vi "AdaptorControl01.vi"() -> ()   [LabVIEW 2011]
panel:
  in  "Local":bool
  in  "stop":bool
  out "Close active":bool
  out "Auto active":bool
  out "Open active":bool
  out "Hold active":bool
  out "Message":string
  out "D active":bool
  out "A active":bool
  out "B active":bool
  out "C active":bool
  in  "v":bool
  in  "^":bool
  in  "Mode":bool
  in  "Zero":bool
  out "Angle":string
  out "Pressure":string
  in  "D":bool
  in  "C":bool
  in  "B":bool
  in  "A":bool
  in  "Close":bool
  in  "Hold":bool
  in  "Open":bool
  in  "Auto":bool
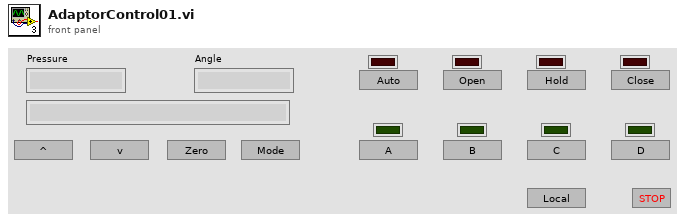
[diagram p1: front panel]
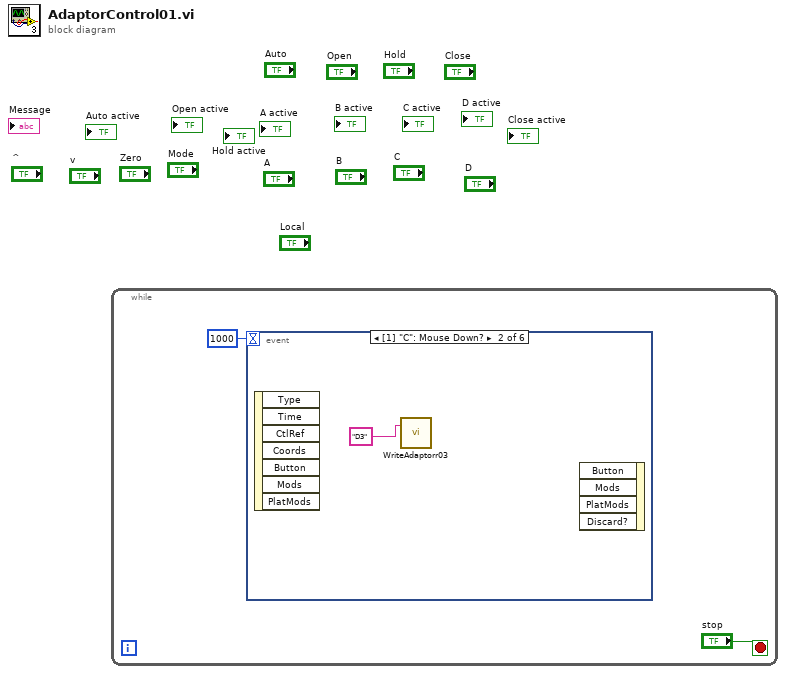
[diagram p0: block diagram]
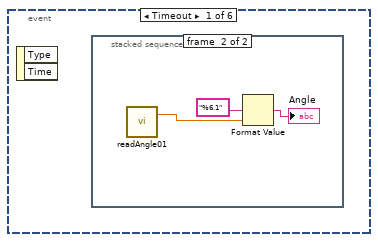
[diagram p2: hidden frame]
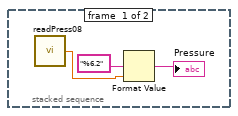
[diagram p3: hidden frame]
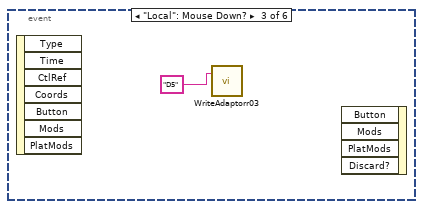
[diagram p4: hidden frame]
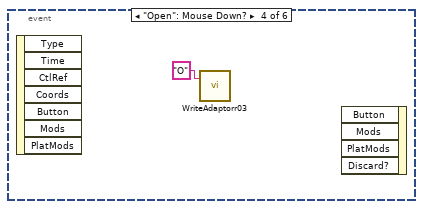
[diagram p5: hidden frame]
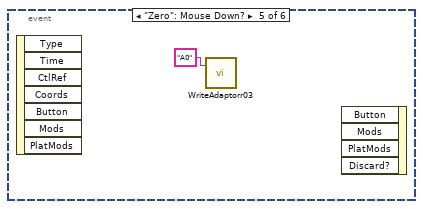
[diagram p6: hidden frame]
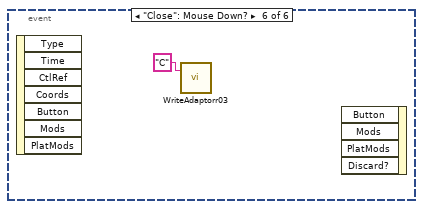
[diagram p7: hidden frame]
diagram:
  n1 = while {
    stop <- "stop" stop-if-true
    n2 = event shown="[1] \"C\": Mouse Down?" {
      selector: _ -> [_ _ _ _ _ _]
      dyn-events: _ -> [_ _ _ _ _ _]
      timeout: 1000 -> [_ _ _ _ _ _]
      event Timeout {
        n3 = event-data() -> ()  [unwired: 1 in, 2 out]
        n4 = stacked-sequence {
          frame #0 {
            n5 = call "readPress08.vi"() -> ("P"=w4:dbl)
            n6 = Format Value(format string="%6.2", value (0)=w4) -> (output string=→"Pressure":string)  [unwired: 1 in]
          }
          frame #1 {
            n7 = call "readAngle01.vi"() -> ("angle"=w6:dbl)  [unwired: 1 in, 1 out]
            n8 = Format Value(format string="%6.1", value (0)=w6) -> (output string=→"Angle":string)  [unwired: 1 in]
          }
        }
      }
      event "C": Mouse Down? {
        n9 = event-data() -> ()  [unwired: 1 in, 7 out]
        n10 = call "WriteAdaptorr03.vi"("string to write"="D3") -> ()  [unwired: 1 in, 1 out]
        n11 = event-data() -> ()  [unwired: 5 in, 1 out]
      }
      event "Local": Mouse Down? {
        n12 = event-data() -> ()  [unwired: 1 in, 7 out]
        n13 = call "WriteAdaptorr03.vi"("string to write"="D5") -> ()  [unwired: 1 in, 1 out]
        n14 = event-data() -> ()  [unwired: 5 in, 1 out]
      }
      event "Open": Mouse Down? {
        n15 = event-data() -> ()  [unwired: 1 in, 7 out]
        n16 = call "WriteAdaptorr03.vi"("string to write"="O") -> ()  [unwired: 1 in, 1 out]
        n17 = event-data() -> ()  [unwired: 5 in, 1 out]
      }
      event "Zero": Mouse Down? {
        n18 = event-data() -> ()  [unwired: 1 in, 7 out]
        n19 = call "WriteAdaptorr03.vi"("string to write"="A0") -> ()  [unwired: 1 in, 1 out]
        n20 = event-data() -> ()  [unwired: 5 in, 1 out]
      }
      event "Close": Mouse Down? {
        n21 = event-data() -> ()  [unwired: 1 in, 7 out]
        n22 = call "WriteAdaptorr03.vi"("string to write"="C") -> ()  [unwired: 1 in, 1 out]
        n23 = event-data() -> ()  [unwired: 5 in, 1 out]
      }
    }
  }
